vi "RequestControlForced.vi"(8 "error in (no error)":errorcluster, 9 "level in":T1, 10 "locked by":string, 11 "BME_DG_System in":refnum<class "BME_DG_System.lvclass">) -> (0 "error out":errorcluster, 1 "level out":T1, 2 "locked by out":string, 3 "BME_DG_System out":refnum<class "BME_DG_System.lvclass">, 5 "Success?":bool)   [LabVIEW 2009, in "POLARIS BME DG.lvlib" / "BME_DG_System.lvclass"]
uses:
  BME_DG_System.lvclass
  ControlLevel.ctl
  BME_DG_System.lvclass/BME_DG_System.ctl
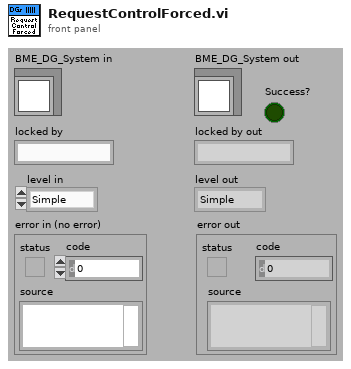
[diagram p1: front panel]
types:
  T1 = typedef "POLARIS BME DG.lvlib/BME_DG_System.lvclass/ControlLevel.ctl" = enum16{"Simple", "Expert", "Unknown"}
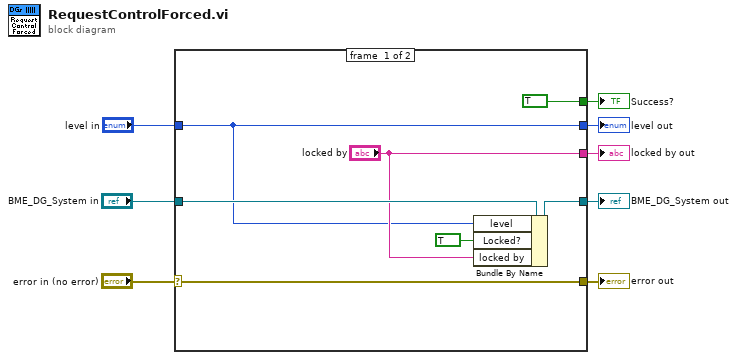
[diagram p0: block diagram]
diagram:
  n1 = case shown="No Error" "error in (no error)" {
    selector: "error in (no error)" -> [w15 w17]
    tunnel: [w15 w17] -> w7
    tunnel: [w14 w16] -> w5
    tunnel: "BME_DG_System in" -> [w13 w16]
    tunnel: ["locked by" _] -> w4
    tunnel: [TRUE _] -> w3
    tunnel: [w10 _] -> w2
    tunnel: "level in" -> [w10 _]
    frame #0 {
      n2 = Bundle By Name(cluster=w13, "level"=w10, "Locked?"=TRUE, "locked by"="locked by") -> (w14:refnum<class "BME_DG_System.lvclass">)
    }
    frame #1 {
    }
  }
  "error out" <- w7
  "BME_DG_System out" <- w5
  "locked by out" <- w4
  "Success?" <- w3
  "level out" <- w2
